vi "AddDebugInfo.vi"(8 "error in (no error)":errorcluster, 9 "ILabVIEWItem":refnum<class "ILabVIEWItem.lvclass">, 11 "CDebugInfo in":refnum<class "CDebugInfo.lvclass">) -> (0 "error out":errorcluster, 3 "CDebugInfo out":refnum<class "CDebugInfo.lvclass">)   [LabVIEW 2020, in "DependencyInspection.lvlib" / "CDebugInfo.lvclass"]
uses:
  CDebugInfo.lvclass
  obj/Addons/LabVIEWObjectInterfaces.lvlibp/LabVIEWObjectInterfaces/ILabVIEWItem/ILabVIEWItem.lvclass
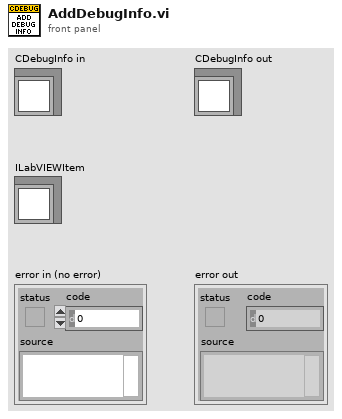
[diagram p1: front panel]
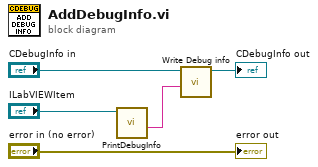
[diagram p0: block diagram]
diagram:
  n1 = call-dynamic "PrintDebugInfo.vi"("ILabVIEWItem in"="ILabVIEWItem") -> ("Debug string"=w1:string)  [unwired: 8 in, 2 out]
  n2 = call-dynamic "Write Debug info.vi"("Debug info"=w1, "CDebugInfo in"="CDebugInfo in") -> ("CDebugInfo out"=→"CDebugInfo out":refnum<class "CDebugInfo.lvclass">)  [unwired: 9 in]
  "error out" <- "error in (no error)"
